vi "IMAQDevice.snap_and_publish.vi"(0 "i ref in":refnum<vi>, 5 "error in (no error)":errorcluster) -> (14 "i ref out":refnum<vi>, 19 "error out":errorcluster)   [LabVIEW 2014, in "IMAQDevice.lvlib"]
doc: "This VI is use in the one-shot mode to capture a picture, which will be saved in the image attribute of the CS class and publish it via DIM. Therefore the picture will be automatically split into several parts so that it can be published.\n\nLicense Agreement for this software:\n\nCopyright (C)\nGesellschaft für Schwerionenforschung, GSI\nPlanckstr. 1\n64291 Darmstadt\nGermany\n\nContact: D.Beck@gsi.de \n\nThis program is free software; you can redistribute it and/or modify it under the terms of the \nGNU General Public License as published by the Free Software Foundation; either version 2 of \nthe license, or (at your option) any later version.\n\nThis program is distributed in the hope that it will be useful, but WITHOUT ANY WARRANTY; \nwithout even the implied warranty of MERCHANTABILITY or FITNESS FOR A PARTICULAR PURPOSE. See the GNU General License for more details (http://www.gnu.org).\n\nGesellschaft für Schwerionenforschung, GSI\nPlanckstr. 1, 64291 Darmstadt, Germany\nFor all questions and ideas contact: M.Richter@gsi.de, H.Brand@gsi.de or D.Beck@gsi.de.\nLast update: 16-JUN-2004"
uses:
  IMAQDevice.lvlib
  CSlibraries-extern/HGF/HGF_LVC/HGF_IMAQ/HGF_IMAQDevice/HGF_IMAQDevice.lvclass
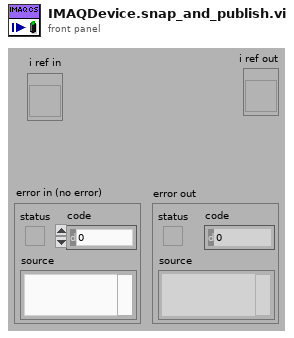
[diagram p1: front panel]
types:
  T1 = typedef "IMAQDevice.lvlib/IMAQDevice.i attribute.ctl" = cluster{"HGF_IMAQ.lvlib:HGF_IMAQDevice.lvclass":refnum<class "HGF_IMAQDevice.lvclass">, "Image":T2, "TimeStampID":i32, "Image IDs":i32[], "NumberOfImagesID":i32, "JPEG?":bool, "JPEGID":i32, "JPEG_ImageID":i32, "TriggerModeID":i32, "OffsetFromLeft":i32, "OffsetFromTop":i32, "HorizontalPixelPerMm":dbl, "VerticalPixelPerMm":dbl, "Grid":cluster{"1":cluster{i32, i32}, "2":cluster{i32, i32}, "3":cluster{i32, i32}, "4":cluster{i32, i32}}, "GridR":cluster{"1":cluster{dbl, dbl}, "2":cluster{dbl, dbl}, "3":cluster{dbl, dbl}, "4":cluster{dbl, dbl}}, "CameraTypeID":i32, "CameraInfos":cluster{"Camera Name-Array":string[], "own Camera Type":string}, "TakeMeasurement?":bool, "TriggerArmedID":i32, "Mirroring":i16, "Rotation":dbl}
  T2 = typedef "IMAQ Image.ctl" = refnum<image>
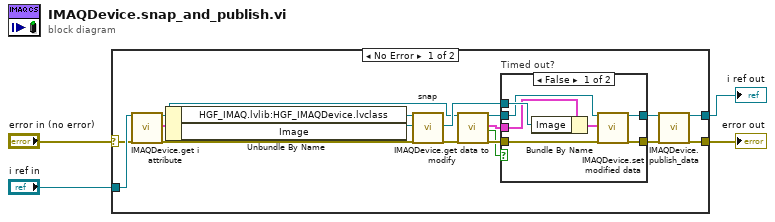
[diagram p0: block diagram]
diagram:
  n1 = case shown="No Error" "error in (no error)" {
    selector: "error in (no error)" -> [w20 w32]
    tunnel: "i ref in" -> [w21 w31]
    tunnel: [w14 w32] -> w2
    tunnel: [w12 w31] -> w1
    frame No Error {
      n2 = call "IMAQDevice.get i attribute.vi"("i ref in"=w21, "error in (no error)"=w20) -> ("i ref out"=w10:refnum<vi>, "i attribute"=w18:T1, "error out"=w17:errorcluster)  [unwired: 15 in]
      n3 = Unbundle By Name(w18) -> ("HGF_IMAQ.lvlib:HGF_IMAQDevice.lvclass"=w16:refnum<class "HGF_IMAQDevice.lvclass">, "Image"=w19:T2)
      n4 = call "snap.vi"("HGF_IMAQDevice"=w16, "Image In"=w19, "error in (no error)"=w17) -> ("Image Out"=w11:T2, "error out"=w6:errorcluster)  [unwired: 14 in, 1 out]
      n5 = call "IMAQDevice.get data to modify.vi"("i ref in"=w10, "error in (no error)"=w6) -> ("i ref out"=w9:refnum<vi>, "i attribute"=w8:T1, "timed out"=w5:bool, "error out"=w7:errorcluster)  [unwired: 14 in]
      n6 = case "Timed out?" shown="False" w5 {
        tunnel: [w27 w29] -> w15
        tunnel: [w26 w30] -> w13
        tunnel: w11 -> [w25 _]
        tunnel: w9 -> [w24 w30]
        tunnel: w8 -> [w23 _]
        tunnel: w7 -> [w22 w29]
        frame False {
          n7 = Bundle By Name(cluster=w23, "Image"=w25) -> (w28:T1)
          n8 = call "IMAQDevice.set modified data.vi"("i ref in"=w24, "i attribute"=w28, "error in (no error)"=w22) -> ("i ref out"=w26:refnum<vi>, "error out"=w27:errorcluster)  [unwired: 15 in]
        }
        frame True {
        }
      }
      n9 = call "IMAQDevice.publish_data.vi"("i ref in"=w13, "error in (no error)"=w15) -> ("i ref out"=w12:refnum<vi>, "error out"=w14:errorcluster)  [unwired: 16 in]
    }
    frame Error {
    }
  }
  "i ref out" <- w1
  "error out" <- w2
